vi "Array To String.vi"(5 "Escape string? [T]":bool=TRUE, 8 "error in (no error)":errorcluster, 10 "Array":string[](array[string]), 11 "Registry Object":refnum<class "Carya Config.lvclass">) -> (0 "error out":errorcluster, 2 "resulting string":string, 3 "Registry Object":refnum<class "Carya Config.lvclass">)   [LabVIEW 2013, in "Carya Config.lvclass"]
doc: "Copyright 2018, Carya Automatisering, Wiebe Walstra."
uses:
  Carya Config.lvclass
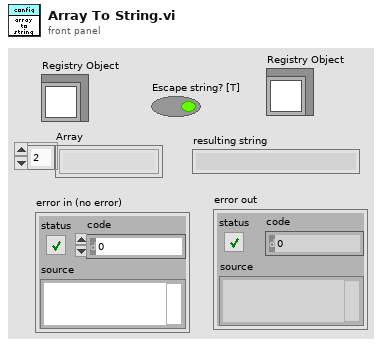
[diagram p1: front panel]
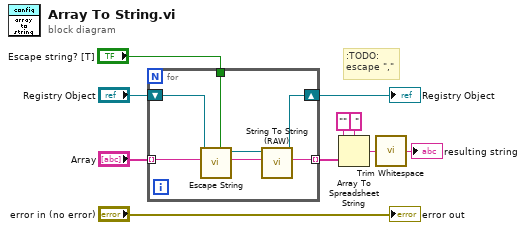
[diagram p0: block diagram]
diagram:
  # ":TODO:\nescape \",\""
  n1 = for {
    tunnel: "Array" -> [w13] mode=indexing
    shift-right: [w17] -> w4
    shift-left: "Registry Object" -> [w15]
    tunnel: [w16] -> w2 mode=indexing
    tunnel: "Escape string? [T]" -> [w11]
    n2 = call-dynamic "Escape String.vi"("Escape string? [T]"=w11, "String"=w13, "Registry Object"=w15) -> ("Escaped string"=w12:string, "Registry Object"=w14:refnum<class "Carya Config.lvclass">)  [unwired: 6 in, 1 out]
    n3 = call-dynamic "String To String (RAW).vi"("String"=w12, "Registry Object"=w14) -> ("String (RAW)"=w16:string, "Registry Object"=w17:refnum<class "Carya Config.lvclass">)  [unwired: 7 in, 1 out]
  }
  "Registry Object" <- w4
  n4 = Array To Spreadsheet String(delimiter (Tab)=", ", array=w2, 3:"" ("format string")) -> (spreadsheet string=w9:string)
  n5 = call <vilib>:"Trim Whitespace.vi"("string"=w9) -> ("trimmed string"=→"resulting string":string)  [unwired: 1 in]
  "error out" <- "error in (no error)"
